vi "zscore.vi"(1 "Array in":dbl[](array[numeric])) -> (0 "Array out":dbl[](array[numeric]))   [LabVIEW 2014]
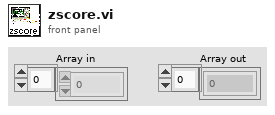
[diagram p1: front panel]
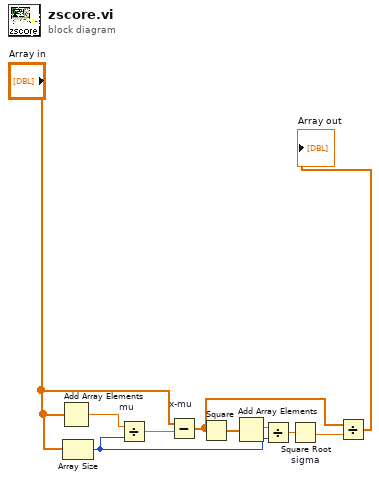
[diagram p0: block diagram]
diagram:
  n1 = Add Array Elements(numeric array="Array in") -> (sum=w1:dbl)
  n2 = Array Size(array="Array in") -> (size(s)=w5:i32)
  n3 = Divide "mu"(x=w1, y=w5) -> (x/y=w2:dbl)
  n4 = Subtract "x-mu"(x="Array in", y=w2) -> (x-y=w9:dbl[])
  n5 = Square(x=w9) -> (x^2=w3:dbl[])
  n6 = Add Array Elements(numeric array=w3) -> (sum=w4:dbl)
  n7 = Divide(x=w4, y=w5) -> (x/y=w6:dbl)
  n8 = Square Root "sigma"(x=w6) -> (sqrt(x)=w8:dbl)
  n9 = Divide(x=w9, y=w8) -> (x/y=→"Array out":dbl[])
